vi "Configure Limiter.vi"(4 "Enable Limiter Beeper (F: Disable)":bool, 6 "Low Limiter Value (-0.3)":dbl=-0.3 min=-15.0 max=15.0 step=0.0001 format="%_4g", 7 "Limiter Value (0.3)":dbl=0.3 min=-15.0 max=15.0 step=1.0 format="%_4g", 8 "error in (no error)":errorcluster, 9 "Enable Separate Setting (F: Disable)":bool, 10 "Source Function  (0: Voltage)":u16(ring) items=["Voltage", "Current"], 11 "VISA resource name":refnum<visa-resource-name>) -> (0 "error out":errorcluster, 3 "VISA resource name out":refnum<visa-resource-name>)   [LabVIEW 2020, in "ADCMT 6240.lvlib"]
doc: "Configure settings of the limiters to prevent damage due to over-voltage or over-current.\nFor a voltage source, the current-limiter is set. For a current-source, the voltage-limiter is set.\nThe limiters for both voltage and current have both HI and LO limiters and they can be set individually.\nFor the voltage-limiter, both HI limiter and LO limiter can set not only bipolar, + /- but also homo-polar, + / +, or -/-."
uses:
  ADCMT 6240.lvlib
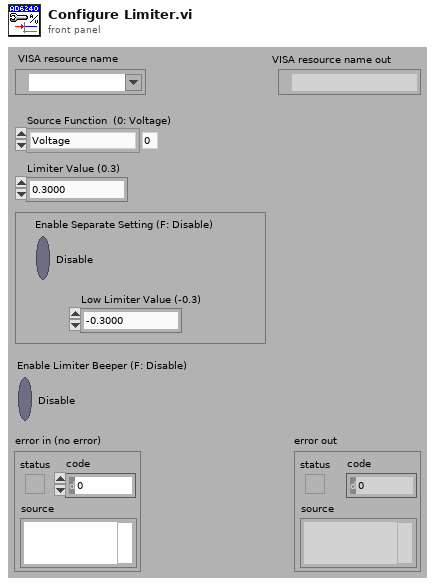
[diagram p1: front panel]
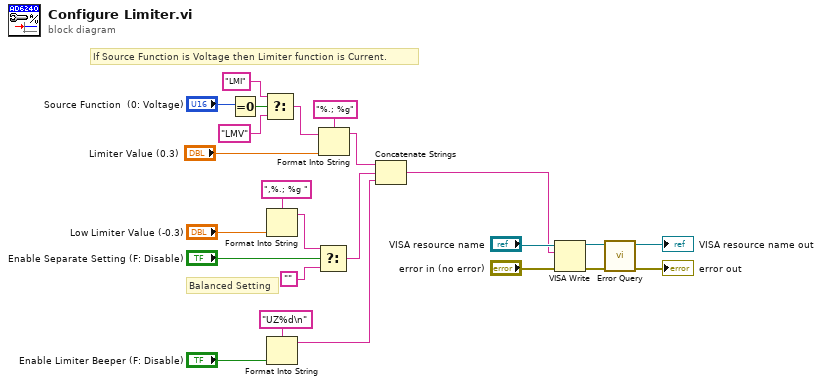
[diagram p0: block diagram]
diagram:
  # "Balanced Setting"
  # "If Source Function is Voltage then Limiter function is Current."
  n1 = Equal To 0?(x="Source Function  (0: Voltage)") -> (x = 0?=w13:bool)
  n2 = Select(t="LMI", s=w13, f="LMV") -> (s? t:f=w10:string)
  n3 = Format Into String(format string=",%.; %g ", "Low Limiter Value (-0.3)") -> (resulting string=w8:string)  [unwired: 2 in, 1 out]
  n4 = Format Into String(format string="UZ%d\n", "Enable Limiter Beeper (F: Disable)") -> (resulting string=w1:string)  [unwired: 2 in, 1 out]
  n5 = Select(t=w8, s="Enable Separate Setting (F: Disable)", f="") -> (s? t:f=w4:string)
  n6 = Format Into String(format string="%.; %g", initial string=w10, "Limiter Value (0.3)") -> (resulting string=w16:string)  [unwired: 1 in, 1 out]
  n7 = Concatenate Strings(w16, w4, w1) -> (w15:string)
  n8 = VISA Write(VISA resource name="VISA resource name", write buffer=w15, error in (no error)="error in (no error)") -> (VISA resource name out=w22:refnum<visa-resource-name>, error out=w21:errorcluster)  [unwired: 1 out]
  n9 = call "Error Query.vi"("error in (no error)"=w21, "VISA resource name"=w22) -> ("error out"=→"error out":errorcluster, "VISA resource name out"=→"VISA resource name out":refnum<visa-resource-name>)  [unwired: 6 in, 2 out]
